vi "Rename String Constants.vi"(8 "error in (no error)":errorcluster, 9 "Replace Strings":string[](array[string]), 10 "Search Strings":string[](array[string]), 11 "vi reference":refnum<vi>) -> (0 "error out":errorcluster, 3 "vi refnum out":refnum<vi>)   [LabVIEW 2020, in "ADAS_IO_Template_MDO.lvclass"]
uses:
  ADAS_IO_Template_MDO.lvclass
  <vilib>/Utility/traverseref.llb/TRef TravTarget.ctl
  <vilib>/Utility/traverseref.llb/VI Scripting - Traverse.lvlib
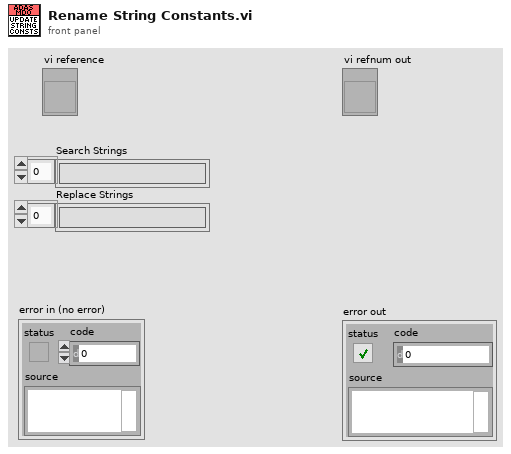
[diagram p1: front panel]
types:
  T1 = enum32{"not a control VI", "control", "typedef", "strict typedef"}
  T2 = typedef "TRef TravTarget.ctl" = enum16{"FP", "BD", "Other"}
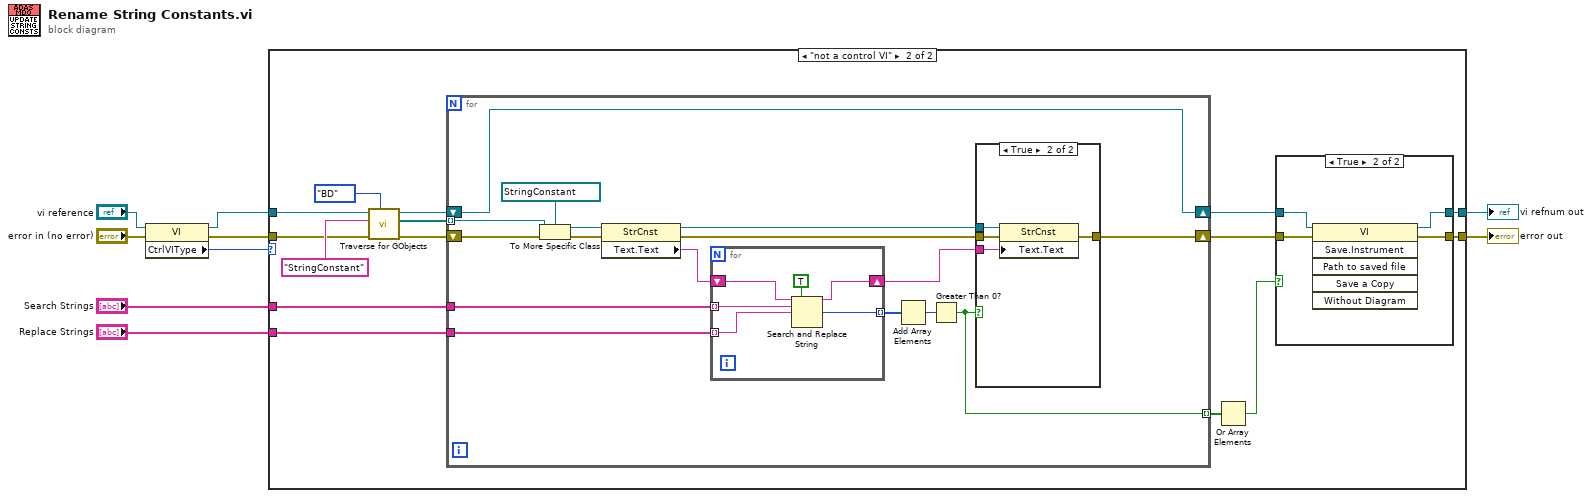
[diagram p0: block diagram]
diagram:
  n1 = property class="VI"(reference="vi reference", error in="error in (no error)") -> (reference out=w2:refnum<vi>, error out=w3:errorcluster, "CtrlVIType"=w1:T1)
  n2 = case shown="\"not a control VI\"" w1 {
    tunnel: "Search Strings" -> [_ w21]
    tunnel: "Replace Strings" -> [_ w20]
    tunnel: [w10 w17] -> w7
    tunnel: [w11 w14] -> w6
    tunnel: w3 -> [w11 w13]
    tunnel: w2 -> [w10 w12]
    frame Default {
    }
    frame "not a control VI" {
      n3 = call <vilib>:"Traverse for GObjects.vi"("Traverse Target"=TRef_TravTarget."BD", "error in (no error)"=w13, "Class Name"="StringConstant", "VI Refnum"=w12) -> ("error out"=w24:errorcluster, "References"=w25:refnum<vi>[], "dup VI Refnum"=w23:refnum<vi>)  [unwired: 4 in, 1 out]
      n4 = for {
        tunnel: w25 -> [w47] mode=indexing
        shift-right: [w33] -> w18
        shift-left: w24 -> [w46]
        shift-right: [w48] -> w19
        shift-left: w23 -> [w48]
        tunnel: w21 -> [w44]
        tunnel: w20 -> [w43]
        tunnel: [w34] -> w16 mode=indexing
        n5 = To More Specific Class(target class=refnum<vi> refnum ("reference"), reference=w47, error in=w46) -> (specific class reference=w41:refnum<vi>, error out=w42:errorcluster)
        n6 = property class="StrCnst"(reference=w41, error in=w42) -> (reference out=w38:refnum<vi>, error out=w37:errorcluster, "Text.Text"=w40:string)
        n7 = for {
          tunnel: w44 -> [w58] mode=indexing
          tunnel: w43 -> [w57] mode=indexing
          shift-right: [w55] -> w36
          shift-left: w40 -> [w56]
          tunnel: [w54] -> w39 mode=indexing
          n8 = Search and Replace String(replace all?=TRUE ("replace all? (F)"), input string=w56, search string=w58, replace string=w57) -> (result string=w55:string, number of replacements=w54:i32)  [unwired: 4 in, 2 out]
        }
        n9 = Add Array Elements(numeric array=w39) -> (sum=w35:i32)
        n10 = Greater Than 0?(x=w35) -> (x > 0?=w34:bool)
        n11 = case shown="True" w34 {
          tunnel: w38 -> [_ w53]
          tunnel: w37 -> [w49 w52]
          tunnel: w36 -> [_ w51]
          tunnel: [w49 w50] -> w33
          frame False {
          }
          frame True {
            n12 = property class="StrCnst"(reference=w53, error in=w52, "Text.Text"=w51) -> (error out=w50:errorcluster)  [unwired: 1 out]
          }
        }
      }
      n13 = Or Array Elements(Boolean array=w16) -> (logical OR=w15:bool)
      n14 = case shown="True" w15 {
        tunnel: w19 -> [w28 w32]
        tunnel: w18 -> [w27 w31]
        tunnel: [w27 w30] -> w14
        tunnel: [w28 w29] -> w17
        frame False {
        }
        frame True {
          n15 = invoke class="VI" method="Save.Instrument"(reference=w32, error in=w31) -> (reference out=w29:refnum<vi>, error out=w30:errorcluster)  [unwired: 4 in, 4 out]
        }
      }
    }
  }
  "error out" <- w6
  "vi refnum out" <- w7
